vi "Arduino_packagePaths.vi"(11 "name":string="33 IoT") -> (3 "String":string)   [LabVIEW 2022 SP3]
panel:
  out "packages":T1(array[cluster])
  out "before substring":string
  out "text 2":string
  out "toolsDependencies":T2(array[cluster])
  out "Options":T3(array[cluster])
  out "text":string
  # "-prefs=runtime.tools.arm-none-eabi-gcc.path=\"PACK/arduino/tools/arm-none-eabi-gcc/7-2017q4\"  -prefs=runtime.tools.arm-none-eabi-gcc.path=\"PACK/arduino/tools/arm-none-eabi-gcc/7-2017q4\"  -prefs=runtime.tools.arduinoOTA.path=\"PACK/arduino/tools/arduinoOTA/1.2.1\" -prefs=runtime.tools.openocd.path=\"PACK/arduino/tools/openocd/0.10.0-arduino7\"  -prefs=runtime.tools.arduinoOTA-1.2.1.path=\"PACK/arduino/tools/arduinoOTA/1.2.1\" -prefs=runtime.tools.openocd-0.10.0-arduino7.path=\"PACK/arduino/tools/openocd/0.10.0-arduino7\""
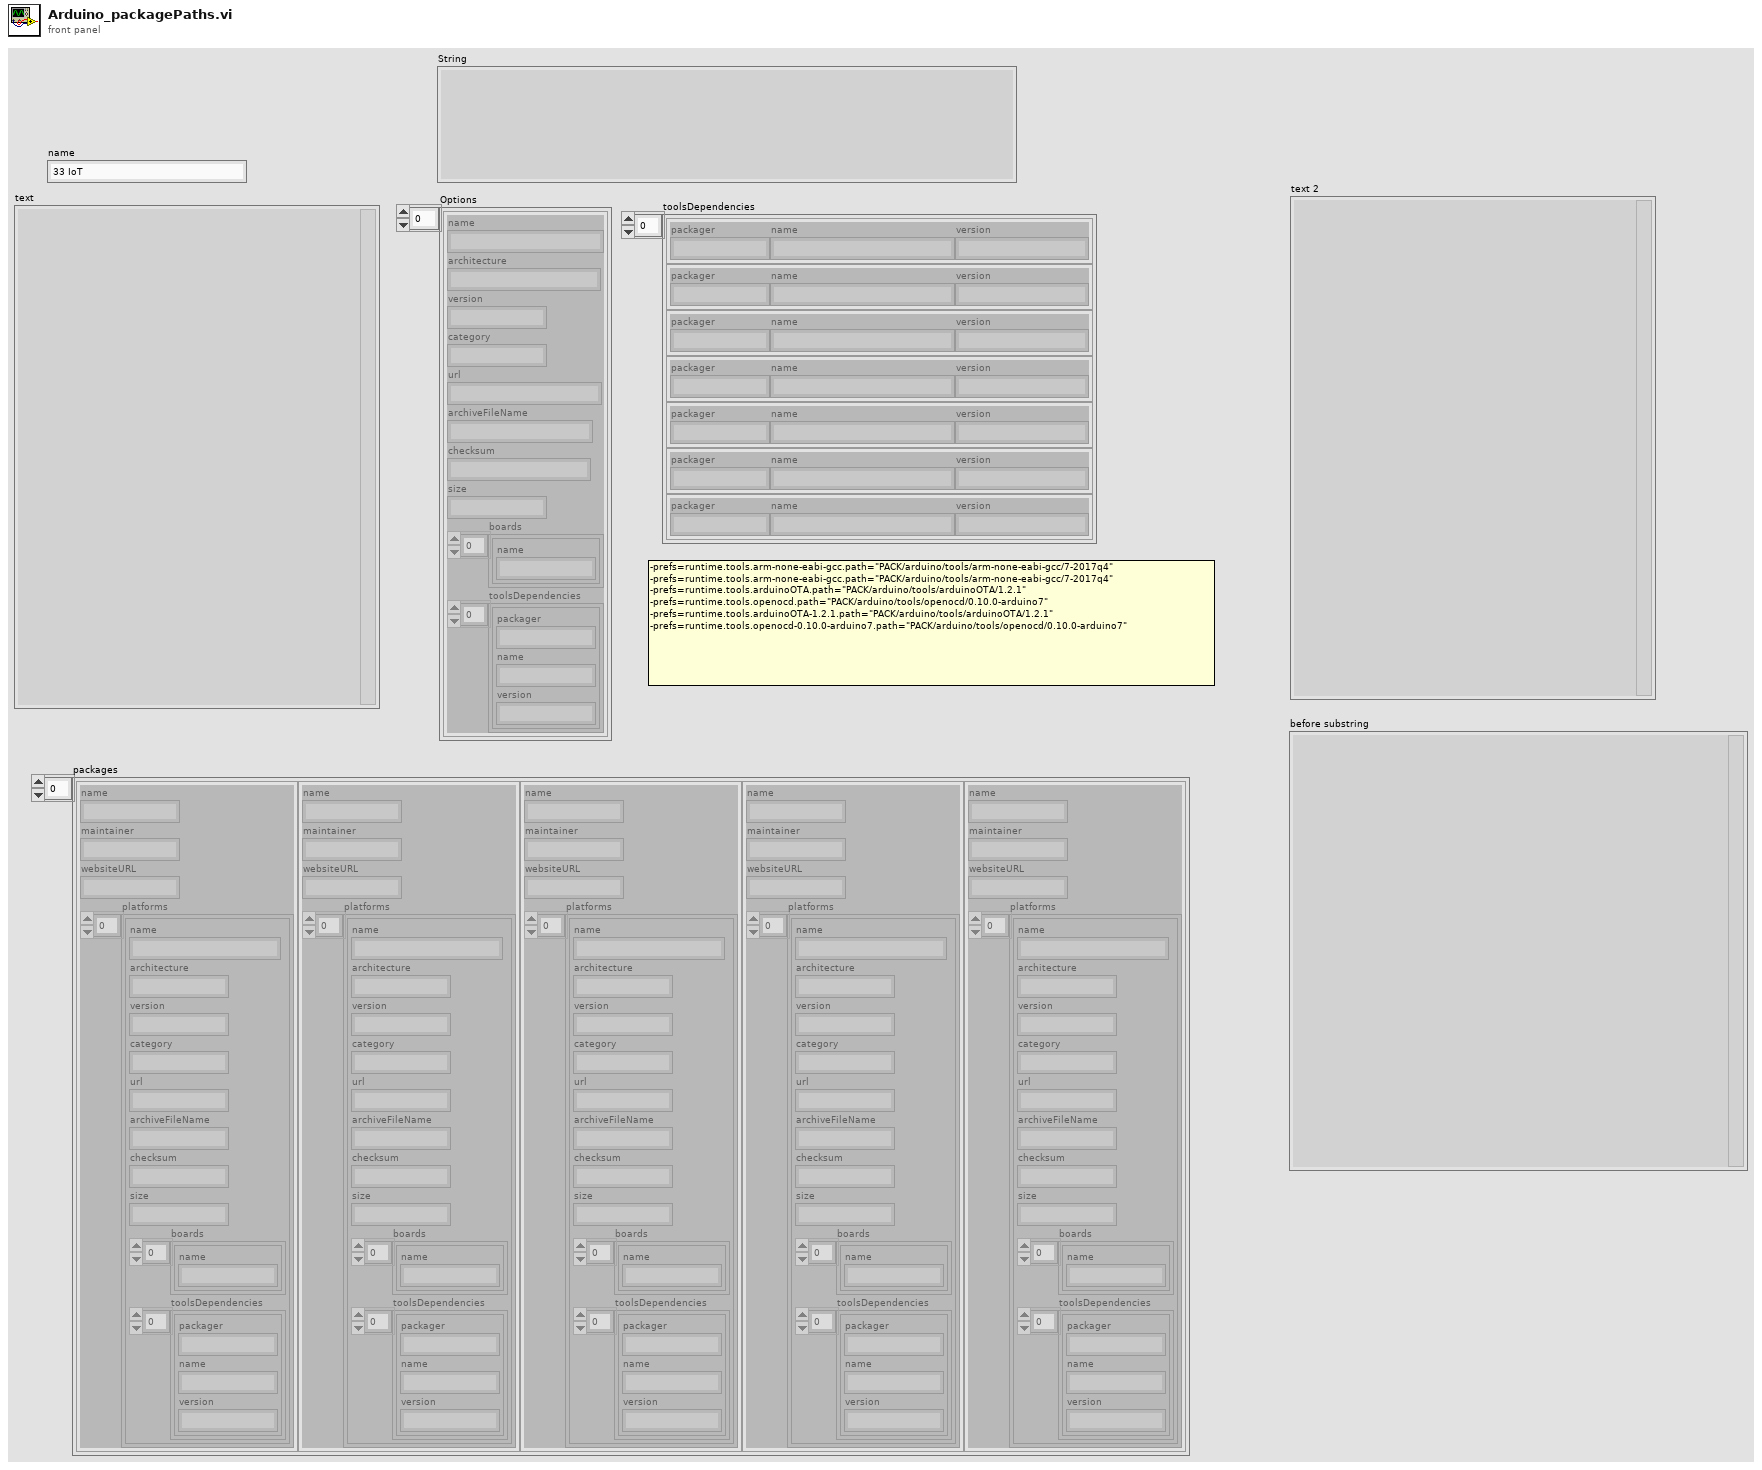
[diagram p1: front panel]
types:
  T1 = cluster{"name":string, "maintainer":string, "websiteURL":string, "platforms":cluster{"name":string, "architecture":string, "version":string, "category":string, "url":string, "archiveFileName":string, "checksum":string, "size":string, "boards":cluster{"name":string}[], "toolsDependencies":cluster{"packager":string, "name":string, "version":string}[]}[]}[]
  T2 = cluster{"packager":string, "name":string, "version":string}[]
  T3 = cluster{"name":string, "architecture":string, "version":string, "category":string, "url":string, "archiveFileName":string, "checksum":string, "size":string, "boards":cluster{"name":string}[], "toolsDependencies":cluster{"packager":string, "name":string, "version":string}[]}[]
  T4 = cluster{"packages":cluster{"name":string, "maintainer":string, "websiteURL":string, "platforms":cluster{"name":string, "architecture":string, "version":string, "category":string, "url":string, "archiveFileName":string, "checksum":string, "size":string, "boards":cluster{"name":string}[], "toolsDependencies":cluster{"packager":string, "name":string, "version":string}[]}[]}[]}
  T5 = cluster{"name":string, "architecture":string, "version":string, "category":string, "url":string, "archiveFileName":string, "checksum":string, "size":string, "boards":cluster{"name":string}[], "toolsDependencies":cluster{"packager":string, "name":string, "version":string}[]}
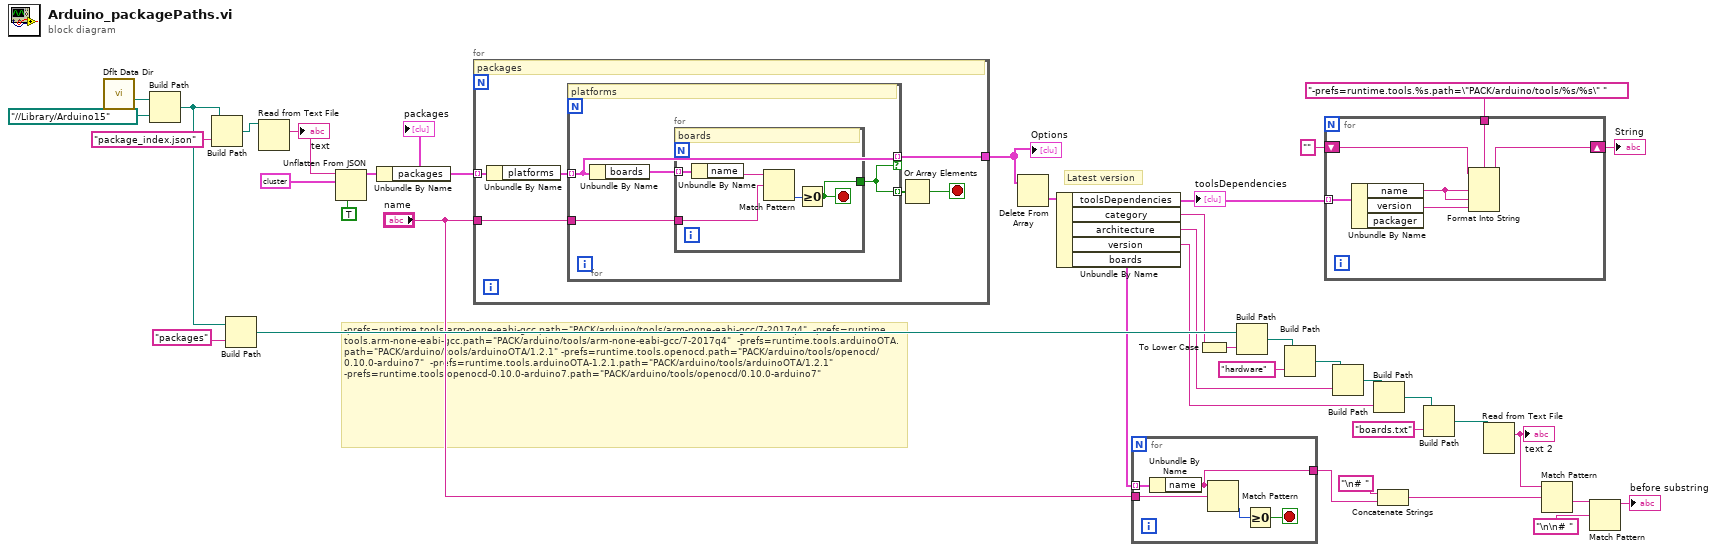
[diagram p0: block diagram]
diagram:
  # "Latest version"
  # "-prefs=runtime.tools.arm-none-eabi-gcc.path=\"PACK/arduino/tools/arm-none-eabi-gcc/7-2017q4\"  -prefs=runtime.tools.arm-none-eabi-gcc.path=\"PACK/arduino/tools/arm-none-eabi-gcc/7-2017q4\"  -prefs=runtime.tools.arduinoOTA.path=\"PACK/arduino/tools/arduinoOTA/1.2.1\" -prefs=runtime.tools.openocd.path=\"PACK/arduino/tools/openocd/0.10.0-arduino7\"  -prefs=runtime.tools.arduinoOTA-1.2.1.path=\"PACK/arduino/tools/arduinoOTA/1.2.1\" -prefs=runtime.tools.openocd-0.10.0-arduino7.path=\"PACK/arduino/tools/openocd/0.10.0-arduino7\""
  n1 = call <vilib>:"Dflt Data Dir.vi"() -> ("App:Default Data Directory"=w38:path)
  n2 = Build Path(base path=w38, name or relative path=path "../../Library/Arduino15") -> (appended path=w23:path)
  n3 = Build Path(base path=w23, name or relative path="package_index.json") -> (appended path=w35:path)
  n4 = Build Path(base path=w23, name or relative path="packages") -> (appended path=w21:path)
  n5 = Read from Text File(file (use dialog)=w35) -> (text=w34:string)  [unwired: 3 in, 3 out]
  "text" <- w34
  n6 = Unflatten From JSON(JSON string=w34, type and defaults=T4 {"packages"=[{"name"="", "maintainer"="", "websiteURL"="", "platforms"=[{"name"=" ", "architecture"="", "version"="", "category"="", "url"="", "archiveFileName"="", "checksum"="", "size"="", "boards"=[{"name"=" "}], "toolsDependencies"=[{"packager"=" ", "name"="", "version"=""}]}]}]}, default null elements? (F)=TRUE) -> (value=w31:T4)  [unwired: 4 in, 1 out]
  n7 = Unbundle By Name(w31) -> ("packages"=w30:T1)
  "packages" <- w30
  n8 = for {
    tunnel: w30 -> [w42] mode=indexing
    tunnel: "name" -> [w43]
    tunnel: [w39] -> w24
    stop <- w40 stop-if-true
    # "packages"
    n9 = Unbundle By Name(w42) -> ("platforms"=w44:T3)
    n10 = for {
      tunnel: w44 -> [w46] mode=indexing
      tunnel: w43 -> [w47]
      tunnel: [w46] -> w39 mode=indexing if=w45
      tunnel: [w45] -> w41 mode=indexing
      # "platforms"
      n11 = Unbundle By Name(w46) -> ("boards"=w48:cluster{"name":string}[])
      n12 = for {
        tunnel: w48 -> [w53] mode=indexing
        tunnel: w47 -> [w51]
        tunnel: [w49] -> w45
        stop <- w49 stop-if-true
        # "boards"
        n13 = Unbundle By Name(w53) -> ("name"=w52:string)
        n14 = Match Pattern(string=w52, regular expression=w51) -> (offset past match=w50:i32)  [unwired: 1 in, 3 out]
        n15 = Greater Or Equal To 0?(x=w50) -> (x >= 0?=w49:bool)
      }
    }
    n16 = Or Array Elements(Boolean array=w41) -> (logical OR=w40:bool)
  }
  "Options" <- w24
  n17 = Delete From Array(array=w24) -> (deleted portion=w29:T5)  [unwired: 2 in, 1 out]
  n18 = Unbundle By Name(w29) -> ("toolsDependencies"=w28:T2, "category"=w20:string, "architecture"=w15:string, "version"=w13:string, "boards"=w9:cluster{"name":string}[])
  "toolsDependencies" <- w28
  n19 = for {
    tunnel: w9 -> [w58] mode=indexing
    tunnel: "name" -> [w57]
    tunnel: [w54] -> w7
    stop <- w56 stop-if-true
    n20 = Unbundle By Name(w58) -> ("name"=w54:string)
    n21 = Match Pattern(string=w54, regular expression=w57) -> (offset past match=w55:i32)  [unwired: 1 in, 3 out]
    n22 = Greater Or Equal To 0?(x=w55) -> (x >= 0?=w56:bool)
  }
  n23 = To Lower Case(string=w20) -> (all lower case string=w19:string)
  n24 = Build Path(base path=w21, name or relative path=w19) -> (appended path=w18:path)
  n25 = Build Path(base path=w18, name or relative path="hardware") -> (appended path=w16:path)
  n26 = for {
    tunnel: w28 -> [w64] mode=indexing
    tunnel: "-prefs=runtime.tools.%s.path=\"PACK/arduino/tools/%s/%s\" " ("format string") -> [w63]
    shift-right: [w59] -> w25
    shift-left: "" -> [w60]
    n27 = Unbundle By Name(w64) -> ("name"=w62:string, "version"=w61:string)  [unwired: 1 out]
    n28 = Format Into String(format string=w63, initial string=w60, w62, w62, w61) -> (resulting string=w59:string)  [unwired: 1 in, 1 out]
  }
  "String" <- w25
  n29 = Build Path(base path=w16, name or relative path=w15) -> (appended path=w14:path)
  n30 = Build Path(base path=w14, name or relative path=w13) -> (appended path=w12:path)
  n31 = Concatenate Strings("\n# " ("string"), w7) -> (w4:string)
  n32 = Build Path(base path=w12, name or relative path="boards.txt") -> (appended path=w10:path)
  n33 = Read from Text File(file (use dialog)=w10) -> (text=w5:string)  [unwired: 3 in, 3 out]
  "text 2" <- w5
  n34 = Match Pattern(string=w5, regular expression=w4) -> (after substring=w3:string)  [unwired: 1 in, 3 out]
  n35 = Match Pattern(string=w3, regular expression="\n\n# " ("string")) -> (before substring=→"before substring":string)  [unwired: 1 in, 3 out]
